vi "wait_01.vi"(0 "total wait time (s)":dbl) -> (1 "Wait time remaining (s)":string, 2 "Done":bool)   [LabVIEW 2011]
uses:
  wait_globals.vi
panel:
  out "Total wait time (s)":string
  out "wait time remaining (s)":dbl
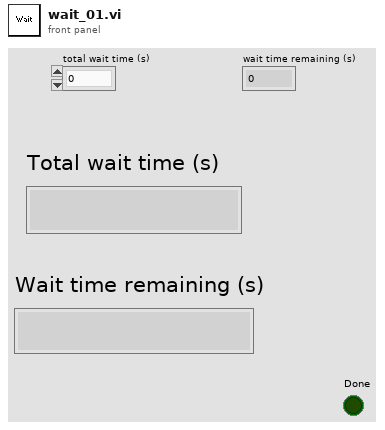
[diagram p1: front panel]
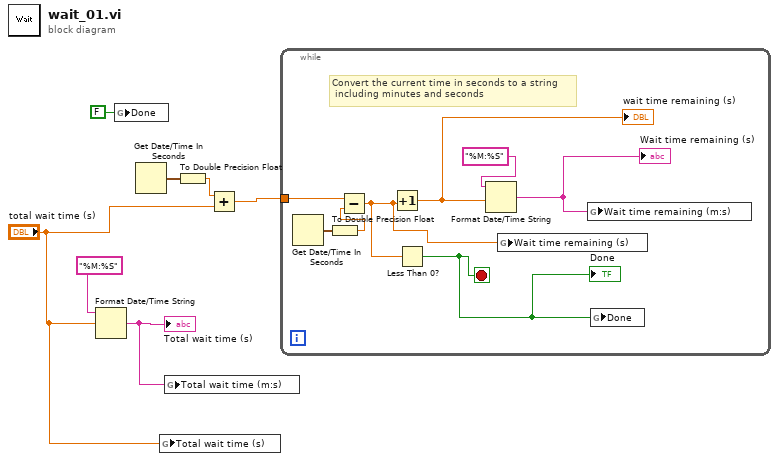
[diagram p0: block diagram]
diagram:
  n1 = Format Date/Time String(time format string (%c)="%M:%S", seconds (now)="total wait time (s)") -> (date/time string=w3:string)  [unwired: 1 out]
  "Total wait time (s)" <- w3
  n2 = global write "wait_globals.vi" "Done"(FALSE ("Done")) -> ()
  n3 = Get Date/Time In Seconds() -> (seconds since 1Jan1904=w6:timestamp)
  n4 = global write "wait_globals.vi" "Total wait time (s)"("total wait time (s)") -> ()
  n5 = global write "wait_globals.vi" "Total wait time (m:s)"(w3) -> ()
  n6 = To Double Precision Float(number=w6) -> (double precision float=w7:dbl)
  n7 = Add(x=w7, y="total wait time (s)") -> (x+y=w5:dbl)
  n8 = while {
    tunnel: w5 -> [w12]
    stop <- w11 stop-if-true
    # "Convert the current time in seconds to a string\n including minutes and seconds"
    n9 = Get Date/Time In Seconds() -> (seconds since 1Jan1904=w13:timestamp)
    n10 = To Double Precision Float(number=w13) -> (double precision float=w14:dbl)
    n11 = Subtract(x=w12, y=w14) -> (x-y=w9:dbl)
    n12 = Increment(x=w9) -> (x+1=w10:dbl)
    "wait time remaining (s)" <- w10
    n13 = Less Than 0?(x=w9) -> (x < 0?=w11:bool)
    "Done" <- w11
    n14 = Format Date/Time String(time format string (%c)="%M:%S", seconds (now)=w10) -> (date/time string=w8:string)  [unwired: 1 out]
    "Wait time remaining (s)" <- w8
    n15 = global write "wait_globals.vi" "Wait time remaining (s)"(w9) -> ()
    n16 = global write "wait_globals.vi" "Wait time remaining (m:s)"(w8) -> ()
    n17 = global write "wait_globals.vi" "Done"(w11) -> ()
  }
